vi "HFRR ADV v10.vi"() -> ()   [LabVIEW 2025]
uses:
  <vilib>/picture/picture.llb/imagedata.ctl
  src/Support Vi/Auto Start enum.ctl
  src/CAMERA CODE/CAMERA LIVE FEED ENUM.ctl
  src/CAMERA CODE/POST ANALYSIS ENUM.ctl
  <vilib>/Utility/NIReport.llb/HTML Report Image Alignment.ctl
  9464fbe3-7a28-44f6-aba5-8c8738b059c4.vi
  65798b11-504e-4bc8-a248-6a605d2bfeff.vi
  e8a7d01f-49de-42c3-94d4-2c8624f58f4e.vi
  5efb8110-29bd-47d9-92d0-c4703c9d257e.vi
  <vilib>/Analysis/baseanly.llb/Mean (DBL).vi
  <vilib>/Analysis/5stat.llb/RMS (DBL).vi
  c311699a-12ba-46ef-ac8f-427021fdbf06.vi
  b1c79803-6f73-4462-b675-f7b5eb88be7c.vi
  62610586-f3e3-47d7-ba3d-7d74a0c80884.vi
  25e8caaf-84ea-468e-9ff7-adb0e8b96af1.vi
  63a25930-3a94-42f5-b8a7-a5485c4ba60b.vi
  865355ac-209e-4fc1-945d-f9c41f79343a.vi
  8bf3357a-fd86-4b15-a53b-ddd460c8ef7b.vi
  8955922f-f541-41b3-8336-ee15e0ce1609.vi
  <vilib>/Analysis/4window.llb/Hanning Window (DBL).vi
  <vilib>/Utility/error.llb/Trim Whitespace One-Sided.vi
  <vilib>/Analysis/4window.llb/AllCosWindow (DBL).vi
  Instance          27 41Saved   WinDucom--std ed hfrr-WO 2464 v02 .vi
  <vilib>/Instr/_visa.llb/VISA Configure Serial Port (Instr).vi
  Instance          17 41Saved   WinDucom--std ed hfrr-WO 2464 v02 .vi
  Instance          37 41Saved   WinDucom--std ed hfrr-WO 2464 v02 .vi
  Instance          15 41Saved   WinDucom--std ed hfrr-WO 2464 v02 .vi
  <vilib>/addons/control/pid/pid.llb/PID (DBL).vi
  Instance          20 41Saved   WinDucom--std ed hfrr-WO 2464 v02 .vi
  <vilib>/measure/matone.llb/Extract Single Tone Information 1 Chan.vi
  Instance          10 41Saved   WinDucom--std ed hfrr-WO 2464 v02 .vi
  Instance          23 41Saved   WinDucom--std ed hfrr-WO 2464 v02 .vi
  <vilib>/Utility/NIReport.llb/Append Image to Report (path wrap).vi
  <vilib>/printing/OpenHTMLReport.llb/Open HTML Report in Browser (Refnum).vi
  <vilib>/Utility/NIReport.llb/Append Report Text (str wrap).vi
  Instance          11 41Saved   WinDucom--std ed hfrr-WO 2464 v02 .vi
  Instance           6 41Saved   WinDucom--std ed hfrr-WO 2464 v02 .vi
  Instance          28 41Saved   WinDucom--std ed hfrr-WO 2464 v02 .vi
  <vilib>/Utility/NIReport.llb/NI_report.lvclass
  <vilib>/addons/control/pid/NI_PID_pid.lvlib
  <vilib>/measure/NI_MAPro.lvlib
  <vilib>/ptbypt/NI_PtbyPt.lvlib
  Instance          22 41Saved   WinDucom--std ed hfrr-WO 2464 v02 .vi
  Instance          25 41Saved   WinDucom--std ed hfrr-WO 2464 v02 .vi
  <vilib>/NI Modbus.llb/MB Serial Master Query Read Input Registers (poly).vi
  Instance          35 41Saved   WinDucom--std ed hfrr-WO 2464 v02 .vi
  Instance          38 41Saved   WinDucom--std ed hfrr-WO 2464 v02 .vi
  <vilib>/measure/NI_MABase.lvlib
  <vilib>/Utility/NIReport.llb/NI_ReportGenerationCore.lvlib
  <vilib>/Analysis/NI_AALPro.lvlib
  <vilib>/Analysis/NI_AALBase.lvlib
  kernel32.dll
  <vilib>/NI Modbus.llb/MB Serial Master Query Write Single Register (poly).vi
panel:
  out "ELAPSED INDICATION":bool
  in  "main tab sub":enum32{"Page 1", "Page 2"}(tab)
  out "About":cluster{"About Display":string}={"About Display"="Software Version : Lab IQ\\WO 2465\\ v10\n\nRelease Period    : April 2026  "}
  in  "Info":bool
  in  "Quit":bool
  out "Humidity Port":bool=TRUE caption="Port 2"
  out "Standard 2":string="ASTM D6079 TEST CONDITIONS"
  out "powstat":bool caption="Power Status"
  out "Test \nStatus":bool caption="Test Status"
  out "Port 3":bool=TRUE caption="Port 1"
  out "Port 1a":bool caption="Port 1 a"
  out "Port 4":bool=TRUE caption="Port 2"
  out "Port 2a":bool caption="Port 2 a"
  in  "Main Dashboard Buttons":T1(radio) caption="Radio Buttons - Customizable"
  out "Time Stamp":string
  in  "Main Tab":T2(tab)
  out "Service Password Log":string="Incorrect Password"
  in  "Password 3":cluster{"Service Password":string}
  in  "Headen Service Button":bool
  in  "Sign In":bool
  in  "USER ID":string
  in  "USERNAME":string
  out "Auto Scar Check":cluster{"String 2":string}
  in  "Calibration":bool
  in  "Auto":bool
  in  "test time":dbl=75.0 caption="TEST DURATION" min=1.0 max=75.0 step=1.0
  in  "Set Rh":dbl=53.0 caption="HUMIDITY" min=53.0 max=53.0 step=1.0
  in  "Set Temp":dbl=60.0 caption="TEMPERATURE" min=40.0 max=150.0 step=1.0
  in  "Set Strk":dbl=1.0 caption="STROKE LENGTH" min=1.0 max=1.0 step=1.0 format="%.3f"
  in  "NORMAL LOAD":dbl=2.0 caption="APPLIED LOAD" min=1.0 max=10.0 step=1.0
  in  "Set Hz":dbl=50.0 caption="FREQUENCY" min=50.0 max=50.0 step=50.0 format="%.1f"
  out "Standard":string="ASTM D6079 TEST CONDITIONS"
  in  "FILE":string caption="FILE NAME"
  in  "Fuel Discription :":string caption="FLUID DESCRIPTION"
  in  "Batch Ref Num :":string caption="BATCH REF NO"
  in  "Remarks :":string caption="REMARKS"
  in  "tested by":string caption="TESTED BY"
  in  "Operator ID":string caption="OPERATOR ID"
  in  "TEST STANDARD":T3(ring)
  in  "Save & Continue":bool
  in  "Calibration 2":enum32{"Main", "Page 2"}(tab)
  in  "Cal Password":string
  out "Wrong Password":string="Wrong Password Entered"
  out "Time Remaining":dbl min=0.0 max=6000.0 step=0.01 format="%<%M:%S>t"
  in  "EVENT LOG":string="4:36:36 PM       Temperature trip enabled\n4:59:03 PM       Test started  — ASTM D6079-25"
  in  "Single/Multiple":enum32{"Single ", "Multiple"}(radio)=enum."Multiple" caption="Radio Buttons - Customizable"
  in  "Single - Graph":u16(ring) items=["Co-efficient of Friction", "Frictional Force ( N )", "ECR ( % )", "Temperature ( Deg C )", "Humidity ( %RH )", "Stroke ( mm )"]
  in  "Num/Graph":enum32{"Numeric Display", "Graph Display"}(radio) caption="Radio Buttons - Customizable"
  in  "Reset Graph":bool
  in  "Main Tab Display":T4(tab)
  in  "FRICVALZ 4":bool
  out "Set Stroke:":dbl
  out "Set Frequency:":dbl
  out "Set Humidity:":dbl
  out "Set Temperature:":dbl
  in  "Humidity":bool
  out "Horizontal Slider Control":dbl(slide) min=0.0 max=100.0 scale=0.0..75.0
  in  "Heater Button":bool
  out "HEATER":bool
  out "Humidity ( %RH )":dbl caption="Humidity 3" format="%.1f"
  out "AIR TEMP":dbl caption="Air Temperature  ( °C )" min=0.0 max=150.0 step=1.0 format="%.1f"
  out "Frequency ( Hz )":dbl=50.0 caption="Frequency" min=10.0 max=250.0 step=0.1 format="%.1f"
  out "Stroke 2":dbl=1.0 caption="Stroke" format="%.3f"
  out "Stroke":dbl=-1.7485910993892546e-16 format="%.3f"
  out "TEMP":dbl min=0.0 max=150.0 step=1.0 format="%.1f"
  out "ecr 3":dbl min=0.0 max=100.0 step=1.0
  out "FF 3":dbl min=0.0 max=12.0 step=0.01 format="%.3f"
  out "COF 3":dbl min=0.0 max=1.0 step=0.001 format="%.3f"
  in  "Ambient Humidity :":dbl format="%.1f"
  out "Hum":dbl=34.66389660208565 min=0.0 max=150.0 step=1.0
  out "Stroke 4":dbl=1.0 caption="Stroke" format="%.3f"
  out "Stroke ( mm )":cluster{"y":dbl, dbl, "y":dbl}(graph) caption="Waveform Chart - Light"
  out "Humidity ( %RH )":dbl(graph) caption="Waveform Chart - Light"
  out "Status 13":bool
  in  "Set Temp 2":dbl=65.0 caption="TRIP" min=20.0 max=150.0 step=1.0
  in  "trip1 8":bool
  in  "FRICVALZ 2":bool
  out "COF 2":dbl min=0.0 max=1.0 step=0.001 format="%.3f"
  out "Coefficient of Friction":dbl(graph) caption="Waveform Chart - Light"
  out "ecr":dbl min=0.0 max=100.0 step=1.0
  out "Electrical Contact Resistance ( % )":dbl(graph) caption="Waveform Chart - Light"
  out "FF 2":dbl min=0.0 max=12.0 step=0.01 format="%.3f"
  out "Frictional Force ( N )":dbl(graph) caption="Waveform Chart - Light"
  out "TEMP 2":dbl=34.66389660208565 min=0.0 max=150.0 step=1.0
  out "Temperature ( Deg C )":dbl(graph) caption="Waveform Chart - Light"
  out "Single":T5(tab)
  out "COF 4":dbl min=0.0 max=1.0 step=0.001 format="%.3f"
  out "Coefficient of Friction":dbl(graph) caption="Waveform Chart - Light"
  out "FF 4":dbl min=0.0 max=12.0 step=0.01 format="%.3f"
  in  "FRICVALZ 3":bool
  out "Frictional Force ( N )":dbl(graph) caption="Waveform Chart - Light"
  out "ecr 4":dbl min=0.0 max=100.0 step=1.0
  out "Electrical Contact Resistance ( % )":dbl(graph) caption="Waveform Chart - Light"
  out "TEMP 3":dbl=34.66389660208565 min=0.0 max=150.0 step=1.0
  out "Temperature ( Deg C )":dbl(graph) caption="Waveform Chart - Light"
  out "Hum 2":dbl=34.66389660208565 min=0.0 max=150.0 step=1.0
  out "Humidity ( %RH )":dbl(graph) caption="Waveform Chart - Light"
  out "Stroke 3":dbl=1.0 caption="Stroke" format="%.3f"
  out "Stroke ( mm )":cluster{"y":dbl, dbl, "y":dbl}(graph) caption="Waveform Chart - Light"
  out "Test Duration Display":string
  in  "Test Duration Status":dbl(slide) scale=0.0..100.0
  in  "RUN":bool
  in  "Auto Start Test":bool caption="RUN"
  out "Auto Scar Check  2":cluster{"String 2":string}
  in  "Magnification len live scar":string(combo)="5x" caption="MAGNIFICATION LEVEL"
  in  "FILE 3":string(combo) caption="FILE NAME"
  in  "SCAR MEASURMENT":enum32{"Auto Scar", "Manual Scar"}(radio)=enum."Manual Scar" caption="Radio Buttons - Customizable"
  in  "Cap Live Image":bool caption="Save Image"
  out "Zoom Factore":dbl format="%#.0f"
  in  "OUT":bool
  in  "In":bool
  in  "Confirm Measrurement":bool
  in  "Magnification :":string(combo)="5x"
  in  "Open Image":bool
  in  "Test File List :":string(combo)
  in  "Calibration Tab":enum32{"Measrument", "Calibrate"}(tab)
  out "Major Axis":dbl
  out "Minor Axis":dbl
  out "Average":dbl
  in  "Back Square":bool
  out "10x Gain":dbl
  out "5x Gain":dbl
  in  "Actual (µm)":dbl=1.0 caption="Actual (mm)" format="%.6f"
  out "Measurment (mm)":dbl caption="mm" format="%.3f"
  in  "Save Change":bool caption="Save Cal"
  in  "change Gain":bool
  in  "Calibrate":bool
  in  "Resize Tool":bool
  in  "Fit to Screen Tool":bool
  in  "ROI Color Tool":bool
  in  "Clear ROI Tool":bool
  in  "Rectangle Tool":bool
  in  "Pan Tool":bool
  in  "line tool":bool
  in  "Frequency":bool
  in  "Sample Temperature":bool
  in  "Stroke":bool
  in  "Humidity":bool
  in  "Air Temperature":bool
  in  "Tab Control 2":T6(tab)=enum."Humidity"
  in  "rstv2":bool
  out "Coefficient Of Friction":cluster{dbl[], dbl[]}[](graph)
  out "КОФ1":dbl caption="COF1 :" min=0.0 max=200.0 step=0.1 format="%.3f"
  out "КОФ2":dbl caption="COF2 :" min=0.0 max=200.0 step=0.1 format="%.3f"
  out "КОФ3":dbl caption="COF3 :" min=0.0 max=200.0 step=0.1 format="%.3f"
  out "КОФ4":dbl caption="COF4 :" min=0.0 max=200.0 step=0.1 format="%.3f"
  in  "RSTV1 3":bool
  out "Air Temperature  ( °C )":cluster{dbl[], dbl[]}[](graph)
  in  "RSTV1 2":bool
  out "Humidity ( %RH )":cluster{dbl[], dbl[]}[](graph)
  in  "RSTV1 4":bool
  out "Stroke ( mm )":cluster{dbl[], dbl[]}[](graph)
  out "КОФ2 5":dbl caption="Stroke 4 :" min=0.0 max=200.0 step=0.1 format="%.3f"
  out "КОФ2 4":dbl caption="Stroke 3 :" min=0.0 max=200.0 step=0.1 format="%.3f"
  out "КОФ2 3":dbl caption="Stroke 2 :" min=0.0 max=200.0 step=0.1 format="%.3f"
  out "КОФ2 2":dbl caption="Stroke 1:" min=0.0 max=200.0 step=0.1 format="%.3f"
  out "CP2":dbl=nan min=0.0 max=200.0 step=0.1 format="%.3f"
  out "CP1":dbl=nan min=0.0 max=200.0 step=0.1 format="%.3f"
  in  "RST CP":bool
  out "Sample Temperature ( °C )":cluster{dbl[], dbl[]}[](graph)
  in  "RST CP 2":bool
  out "XY Graph 13":cluster{dbl[], dbl[]}[](graph)
  out "Frequency ( Hz )":cluster{dbl[], dbl[]}[](graph)
  in  "RST CP 3":bool
  out "Air Temp ( °C ) vs Humidity ( % RH )":cluster{dbl[], dbl[]}[](graph)
  in  "OPEN 1":bool
  out "String Control 2":string="  "
  out "String Control":string
  out "String Control 7":string
  in  "OPEN 4":bool
  out "String Control 8":string=" "
  in  "OPEN 2":bool
  out "String Control 3":string
  out "String Control 4":string=" "
  in  "OPEN 3":bool
  out "String Control 6":string=" "
  out "String Control 5":string
  in  "Coefficient Of Friction":bool
  in  "OPEN":bool
  in  "Tab Control 5":T7(tab)
  in  "message":string="*Entered password is wrong"
  in  "Password 2":string caption="Password (Advance Setting)"
  in  "EDIT 2":bool
  in  "Language Selection":enum16{"English", "Russian"}(ring)
  in  "SrvM CP 2":bool caption="Reset calibrate\n password"
  in  "SrvM CP":bool caption="Reset calibrate\n password"
  in  "Password":string
  in  "SAVE":bool
  in  "File Path":path=path "C:/LAB-IQ-NXT 2010/1582/1582" caption="File path"
  in  "EDIT":bool
  out "AIR TEMPERATURE  Calibration Error":dbl=1.0 caption="Air Temperature :" min=0.0001 max=100.0 step=0.0001
  out "TEMPERATURE  Calibration Error":dbl=1.0 caption="Temperature :" min=0.0001 max=100.0 step=0.0001
  out "HUMIDITY  Calibration Error":dbl=1.0 caption="Humidity :"
  out "DISPLACEMENT  Calibration Error":dbl=1.0255 caption="Displacement :"
  out "STROKE Calibration Error":dbl=700.0 caption="Stroke Gain :"
  out "FRIC. FORCE Calibration Error":dbl=3.7633 caption="Frictional Force :" min=0.0001 max=100.0 step=0.0001
  in  "AIR TEMP INTERCEPT: 2":dbl=-2.9906 caption="Air Temperature Intercept:" format="%.4f"
  in  "AIR TEMP INTERCEPT:":dbl caption="Air Temperature Intercept :" format="%.4f"
  in  "TEMP INTERCEPT: 2":dbl=-2.9906 caption="Temperature Intercept :" format="%.4f"
  in  "TEMP INTERCEPT:":dbl caption="Temperature Intercept :" format="%.4f"
  in  "AIR TEMPERATURE : 2":dbl=57.9984 caption="Air Temperature :" min=0.0001 max=100.0 step=0.0001 format="%.4f"
  in  "AIR TEMPERATURE :":dbl=1.0 caption="Air Temperature :" min=0.0001 max=100.0 step=0.0001 format="%.4f"
  in  "TEMPERATURE : 2":dbl=57.9984 caption="Temperature :" min=0.0001 max=100.0 step=0.0001 format="%.4f"
  in  "TEMPERATURE :":dbl=1.0 caption="Temperature :" min=0.0001 max=100.0 step=0.0001 format="%.4f"
  in  "HUMIDITY: 2":dbl=1.0 caption="Humidity :" min=0.95 max=1.05 step=0.001 format="%.2f"
  in  "HUMIDITY:":dbl=1.0 caption="Humidity :" min=0.95 max=1.05 step=0.01 format="%.2f"
  in  "DISPLACEMENT : 4":dbl=0.88 caption="Displacement :" min=0.5 max=1.8 step=0.01 format="%#.2f"
  in  "DISPLACEMENT :":dbl=1.0255 caption="Displacement :"
  in  "STROKE GAIN : 2":dbl=900.0 caption="Stroke Gain :" min=500.0 max=1500.0 format="%#.1f"
  in  "STROKE GAIN :":dbl=700.0 caption="Stroke Gain :"
  in  "FRIC. FORCE : 2":dbl=1.0 caption="Frictional Force :" min=0.95 max=1.05 step=0.0001 format="%.2f"
  in  "FRIC. FORCE :":dbl=3.7633 caption="Frictional Force :" min=0.0001 max=100.0 step=0.0001 format="%.4f"
  in  "Tab Control 7":T8(tab)
  out "software msrnt 2":dbl=50.0 caption="Sensor measurment" min=0.0 max=250.0 step=0.001 format="%.4f"
  in  "S.NO":string="1333"
  out "DISPLACEMENT : 3":dbl=1.0255 caption="Corrected  gain:" format="%_2g"
  in  "DISPLACEMENT : 2":dbl=1.0 caption="Displacement  gain:" format="%_3g"
  in  "Standard Slip Gauge (mm)":dbl
  out "String 26":string="Rh"
  out "String 13":string="Rh"
  out "String 5":string="N"
  out "String 3":string="Hz"
  out "Time slide":dbl(slide)=70.0 scale=0.0..2500.0
  in  "Threshold":dbl=0.2 min=0.0 max=5.0 step=0.001 format="%.3f"
  out "Lift":bool
  out "FF Calibration g":dbl[](graph)=[-0.1159806317003227, -0.11422308310659272, -0.10192024295047254, -0.10719288873166506, -0.09840514576301, -0.1036777915442051, -0.09489004857554746, -0.08961740279435236, -0.10192024295047254, -0.09664759716928002, -0.08785985420062238, -0.08785985420062238, -0.08434475701316244, -0.0755570140445048, -0.07204191685704484, -0.07204191685704484, -0.0808296598256999, -0.07379946545077481, -0.07379946545077481, -0.0755570140445048, -0.07379946545077481, -0.07204191685704484, -0.0755570140445048, -0.07028436826331227, -0.07379946545077481, -0.07379946545077481, -0.0685268196695823, 0.014077964235786087, -0.02458810482629926, -0.05270888232599699, -0.0632541738883872, -0.059739076700924654, -0.07379946545077481, -0.0755570140445048, -0.06501172248211717, -0.0685268196695823, -0.06501172248211717, -0.0632541738883872, -0.07028436826331227, -0.06501172248211717, -0.06149662529465463, -0.05622397951346211, -0.05622397951346211, -0.05622397951346211, -0.054466430919732134, -0.054466430919732134, -0.04919378513853445, -0.04392113935734194, -0.04743623654480447, -0.04392113935734194, -0.04392113935734194, -0.03689094498241944, -0.028103202013764383, -0.02107300763883672, -0.02107300763883672, -0.017557910451374184, -0.017557910451374184, -0.010527716076451686, -0.008770167482716543, -0.008770167482716543, -0.008770167482716543, -0.007012618888986565, -0.0017399731077940475, 0.001775124079668492, 0.007047769860861009, 0.012320415642053526, 0.019350610016981188, 0.029895901579366224, 0.036926095954293886, 0.033410998766831346, 0.033410998766831346, 0.036926095954293886, 0.04395629032921638, 0.05098648470414146, 0.05625913048533398, 0.06504687345399161, 0.06856197064145415, 0.0773497136101118, 0.09316765095369194, 0.08789500517249683, 0.09844029673488704, 0.10195539392234698, 0.10722803970354466, 0.11074313689100462, 0.11425823407846716, 0.11425823407846716, 0.12656107423458476, 0.1353488172032424, 0.14413656017189747, 0.1546818517342851, 0.16171204610921017, 0.16874224048413264, 0.1652271432966701, 0.1757724348590603, 0.17752998345279028, 0.18983282360890788, 0.18983282360890788, 0.19862056657756552, 0.20389321235875804, 0.21092340673368312, 0.22146869829607074, 0.22674134407726326, 0.22146869829607074, 0.22498379548353328, 0.2302564412647258, 0.2355290870459209, 0.24080173282711342, 0.24783192720204109, 0.24783192720204109, 0.254862121576961, 0.26189231595188867, 0.26892251032681375, 0.26892251032681375, 0.27419515610800627, 0.2777102532954714, 0.28474044767039386, 0.2900130934515864, 0.29177064204532155, 0.30758857938889905, 0.3058310307951691, 0.3128612251700916, 0.3251640653262118, 0.3234065167324818, 0.33746690548233194, 0.3304367111074043, 0.335709356888602, 0.41304149501277265, 0.3603150372008346, 0.35679994001337206, 0.35504239141964206, 0.3638301343882997, 0.36734523157576227, 0.4165565922002352, 0.45698020985605314, 0.4710405986059007, 0.47279814719963065, 0.4815858901682883, 0.4833434387620183, 0.5114642162617212, 0.4938887303244085, 0.4235867865751603, 0.39546600907546, 0.3884358147005323, 0.3884358147005323, 0.38667826610680234, 0.3919509118879974, 0.39546600907546, 0.4007386548566525, 0.3989811062629225, 0.4007386548566525, 0.40601130063784757, 0.40776884923158013, 0.4112839464190401, 0.4183141407939652, 0.42007168938769773, 0.42534433516889286, 0.4306169809500828, 0.43764717532500785, 0.44467736969993293, 0.4552226612623206, 0.4552226612623206, 0.4552226612623206, 0.4552226612623206, 0.45698020985605314, 0.4657679528247108, 0.4587377584497831, 0.45698020985605314, 0.4622528556372482, 0.4604953070435131, 0.4587377584497831, 0.47279814719963065, 0.4640104042309782, 0.4657679528247108, 0.46928305001217074, 0.4780707929808258, 0.4780707929808258, 0.47631324438709577, 0.4780707929808258, 0.47982834157455834, 0.48510098735575086, 0.49037363313694593, 0.49213118173067594, 0.49564627891813845, 0.5061915704805287, 0.5079491190742587, 0.5184944106366437, 0.5167368620429111, 0.5114642162617212, 0.5097066676679887, 0.5149793134491786, 0.5079491190742587, 0.5114642162617212, 0.5132217648554511, 0.5149793134491786, 0.5202519592303763, 0.5202519592303763, 0.5255246050115687, 0.5272821536053013, 0.5272821536053013, 0.5395849937614215, 0.536069896573959, 0.536069896573959, 0.5395849937614215, 0.5395849937614215, 0.5431000909488815, 0.5431000909488815, 0.5483727367300766, 0.553645382511269, 0.5501302853238066, 0.5483727367300766, 0.5483727367300766, 0.5518878339175392, 0.5501302853238066, 0.5501302853238066, 0.5606755768861942, 0.5571604796987316, 0.5641906740736593, 0.5589180282924616, 0.5571604796987316, 0.553645382511269, 0.5554029311050016, 0.5571604796987316, 0.5641906740736593, 0.5659482226673893, 0.5659482226673893, 0.5659482226673893, 0.5659482226673893, 0.5729784170423143, 0.5764935142297769, 0.5782510628235095, 0.5747359656360443, 0.5800086114172394, 0.5782510628235095, 0.5782510628235095, 0.5764935142297769, 0.5817661600109719, 0.5852812571984319, 0.592311451573357, 0.5993416459482795, 0.6098869375106697, 0.696006818603498, 0.7223700475094658, 0.6397652636040975, 0.6327350692291749, 0.6221897776667898, 0.6221897776667898, 0.6274624234479824, 0.6221897776667898, 0.6327350692291749, 0.6380077150103675, 0.6432803607915599, 0.64152281219783, 0.64152281219783, 0.6520681037602176, 0.6590982981351426, 0.6590982981351426, 0.6573407495414101, 0.6573407495414101, 0.6590982981351426, 0.6608558467288727, 0.6696435896975302, 0.6573407495414101, 0.6608558467288727, 0.6696435896975302, 0.6714011382912628, 0.6731586868849928, 0.6766737840724554, 0.6801888812599153, 0.6784313326661854, 0.6766737840724554, 0.6819464298536478, 0.6784313326661854, 0.6784313326661854, 0.6749162354787203, 0.6749162354787203, 0.6749162354787203, 0.6749162354787203, 0.6784313326661854, 0.6837039784473778, 0.6819464298536478, 0.6819464298536478, 0.6854615270411104, 0.6837039784473778, 0.6784313326661854, 0.6784313326661854, 0.6749162354787203, 0.6784313326661854, 0.6784313326661854, 0.6714011382912628, 0.6696435896975302, 0.6696435896975302, 0.6626133953226078, 0.6714011382912628, 0.6608558467288727, 0.6538256523539502, 0.6520681037602176, 0.6538256523539502, 0.6503105551664876, 0.6555832009476801, 0.6590982981351426, 0.6626133953226078, 0.6643709439163378, 0.6608558467288727, 0.6590982981351426, 0.6520681037602176, 0.6432803607915599, 0.6432803607915599, 0.6538256523539502, 0.6467954579790225, 0.6450379093852925, 0.6450379093852925, 0.6450379093852925, 0.64152281219783, 0.6432803607915599, 0.64152281219783, 0.6380077150103675, 0.6362501664166375, 0.6344926178229049, 0.6344926178229049, 0.6362501664166375, 0.6362501664166375, 0.64152281219783, 0.6432803607915599, 0.6450379093852925, 0.6520681037602176, 0.6520681037602176, 0.648553006572755, 0.6538256523539502, 0.6538256523539502, 0.6590982981351426, 0.6643709439163378, 0.6696435896975302, 0.6837039784473778, 0.6872190756348404, 0.6924917214160355, 0.697764367197228, 0.6924917214160355, 0.6942492700097681, 0.7100672073533482, 0.7698238595402062, 0.7311577904781209, 0.7223700475094658, 0.7223700475094658, 0.7241275961031958, 0.7294002418843883, 0.7733389567276687, 0.8330956089145345, 0.8278229631333368, 0.8418833518831895, 0.8506710948518446, 0.8664890321954247, 0.8717616779766173, 0.8893371639139299, 0.9016400040700475, 0.9121852956324352, 0.9280032329760178, 0.9139428442261678, 0.9139428442261678, 0.9157003928198977, 0.9227305871948254, 0.9543664618819856, 0.9561240104757156, 0.9420636217258654, 0.9789721421942235, 0.9543664618819856, 0.9666693020381032, 0.980729690787956, 0.9666693020381032, 0.892852261101395, 0.8787918723515449, 0.8840645181327375, 0.8823069695390074, 0.8858220667264675, 0.8875796153202, 0.8875796153202, 0.8840645181327375, 0.8893371639139299, 0.8893371639139299, 0.8981249068825851, 0.8981249068825851, 0.8981249068825851, 0.8981249068825851, 0.9051551012575126, 0.9051551012575126, 0.9192154900073628, 0.9104277470387052, 0.9139428442261678, 0.9192154900073628, 0.9244881357885554, 0.9227305871948254, 0.9209730386010928, 0.9280032329760178, 0.9297607815697478, 0.933275878757213, 0.9367909759446755, 0.9385485245384029, 0.9367909759446755, 0.9403060731321329, 0.9438211703195954, 0.9543664618819856, 0.9420636217258654, 0.9473362675070606, 0.9473362675070606, 0.9490938161007906, 0.9490938161007906, 0.9473362675070606, 0.9473362675070606, 0.9508513646945231, 0.9543664618819856, 0.9596391076631782, 0.9578815590694456, 0.9613966562569107, 0.9631542048506433, 0.9719419478192983, 0.9754570450067583, 0.980729690787956, 0.9877598851628785, 0.9877598851628785, 0.9877598851628785, 0.9947900795378062, 0.9965476281315361, 0.9912749823503436, 0.989517433756611, 0.9983051767252686, 1.0018202739127287, 1.0053353711001938, 1.0088504682876562, 1.0123655654751162, 1.0211533084437738, 1.0158806626625763, 1.0193957598500414, 1.0281835028186963, 1.0229108570375038, 1.0246684056312338, 1.0281835028186963, 1.0281835028186963, 1.0281835028186963, 1.035213697193624, 1.035213697193624, 1.0369712457873541, 1.0334561485998914, 1.0404863429748166, 1.045758988756009, 1.0369712457873541, 1.0334561485998914, 1.0404863429748166, 1.031698600006159, 1.0334561485998914, 1.0387287943810866, 1.0404863429748166, 1.0422438915685466, 1.044001440162279, 1.1195760296927224, 1.1371515156300351, 1.0580618289121266, 1.0510316345372042, 1.0387287943810866, 1.0387287943810866, 1.0369712457873541, 1.031698600006159, 1.0404863429748166, 1.0404863429748166, 1.044001440162279, 1.045758988756009, 1.045758988756009, 1.045758988756009, 1.0510316345372042, 1.045758988756009, 1.0422438915685466, 1.0422438915685466, 1.0387287943810866, 1.0334561485998914, 1.0369712457873541, 1.0387287943810866, 1.031698600006159, 1.0387287943810866, 1.029941051412429, 1.0404863429748166, 1.031698600006159, 1.0334561485998914, 1.035213697193624, 1.0369712457873541, 1.0334561485998914, 1.0334561485998914, 1.0527891831309368, 1.0422438915685466, 1.035213697193624, 1.0334561485998914, 1.029941051412429, 1.0264259542249663, 1.0281835028186963, 1.0211533084437738, 1.0264259542249663, 1.0158806626625763, 1.0158806626625763, 1.0176382112563087, 1.0106080168813836, 1.0088504682876562, 1.0088504682876562, 1.0070929196939262, 1.0070929196939262, 1.0123655654751162, 1.0123655654751162, 1.0158806626625763, 1.0158806626625763, 1.0176382112563087, 1.0229108570375038, 1.0141231140688463, 1.0158806626625763, 1.0193957598500414, 1.0176382112563087, 1.0176382112563087, 1.0193957598500414, 1.0229108570375038, 1.0264259542249663, 1.0229108570375038, 1.031698600006159, 1.0264259542249663, 1.0334561485998914, 1.0369712457873541, 1.0422438915685466, 1.0527891831309368, 1.0492740859434742, 1.0492740859434742, 1.0545467317246642, 1.0563042803183942, 1.0615769260995918, 1.0650920232870518, 1.070364669068247, 1.0756373148494394, 1.084425057818097, 1.091455252193022, 1.0949703493804845, 1.102000543755407, 1.1090307381303321, 1.1195760296927224, 1.117818481098987, 1.1230911268801824, 1.1301213212551073, 1.1266062240676449, 1.1248486754739149, 1.1318788698488373, 1.1371515156300351, 1.1512119043798827, 1.1512119043798827, 1.1547270015673425, 1.1599996473485377, 1.1705449389109253, 1.1740600360983877, 1.1723024875046555, 1.175817584692118, 1.179332681879583, 1.2320591396915157, 1.2144836537542059, 1.2426044312539035, 1.2900582432846492, 1.3006035348470342, 1.3076337292219617, 1.3287243123467318, 1.3656328328150897, 1.3691479300025498, 1.37969322156494, 1.3779356729712073, 1.388480964533595, 1.39375361031479, 1.402541353283445, 1.4095715476583677, 1.4130866448458301, 1.4183592906270253, 1.4078139990646377, 1.4166017420332928, 1.402541353283445, 1.4060564504709077, 1.420116839220758, 1.4183592906270253, 1.4113290962521003, 1.4218743878144877, 1.420116839220758, 1.3867234159398627, 1.36739038140882, 1.3621177356276275, 1.3586026384401648, 1.3709054785962824, 1.36739038140882, 1.36739038140882, 1.36739038140882, 1.36739038140882, 1.3656328328150897, 1.36739038140882, 1.3638752842213573, 1.3603601870338946, 1.3515724440652397, 1.3515724440652397, 1.3410271525028519, 1.3375120553153894, 1.332239409534197, 1.3269667637530018, 1.3216941179718094, 1.3234516665655394, 1.309391277815692, 1.2812705003159917, 1.2988459862533042, 1.3252092151592694, 1.3129063750031542, 1.3041186320344993, 1.3041186320344993, 1.3023610834407642, 1.293573340472109, 1.3041186320344993, 1.2953308890658417, 1.2847855975034512, 1.291815791878379, 1.291815791878379, 1.2900582432846492, 1.3006035348470342, 1.288300694690914, 1.2830280489097214, 1.2830280489097214, 1.2847855975034512, 1.2847855975034512, 1.288300694690914, 1.288300694690914, 1.2900582432846492, 1.2900582432846492, 1.291815791878379, 1.2988459862533042, 1.3006035348470342, 1.3006035348470342, 1.293573340472109, 1.288300694690914, 1.2988459862533042, 1.3006035348470342, 1.3023610834407642, 1.3023610834407642, 1.2970884376595715, 1.2953308890658417, 1.3006035348470342, 1.2988459862533042, 1.3006035348470342, 1.3076337292219617, 1.309391277815692, 1.309391277815692, 1.3164214721906167, 1.3287243123467318, 1.3287243123467318, 1.3269667637530018, 1.3287243123467318, 1.3410271525028519, 1.3445422496903146, 1.3515724440652397, 1.3533299926589721, 1.3621177356276275, 1.3621177356276275, 1.3656328328150897, 1.3744205757837422, 1.3744205757837422, 1.3709054785962824, 1.3744205757837422, 1.3761781243774776, 1.3779356729712073, 1.38145077015867, 1.3849658673461325, 1.3902385131273278, 1.3919960617210576, 1.3902385131273278, 1.4253894850019504, 1.420116839220758, 1.3304818609404645, 1.3146639235968844, 1.3146639235968844, 1.3129063750031542, 1.3146639235968844, 1.318179020784347, 1.318179020784347, 1.3216941179718094, 1.3252092151592694, 1.332239409534197, 1.3304818609404645, 1.3252092151592694, 1.3252092151592694, 1.319936569378077, 1.3216941179718094, 1.3216941179718094, 1.3216941179718094, 1.319936569378077, 1.319936569378077, 1.319936569378077, 1.318179020784347, 1.3146639235968844, 1.3234516665655394, 1.319936569378077, 1.3164214721906167, 1.3216941179718094, 1.319936569378077, 1.3146639235968844, 1.3164214721906167, 1.3164214721906167, 1.3164214721906167, 1.3357545067216594, 1.318179020784347, 1.3146639235968844, 1.3129063750031542, 1.3058761806282293, 1.3111488264094218, 1.3058761806282293, 1.3076337292219617, 1.3216941179718094, 1.3146639235968844, 1.3146639235968844, 1.3111488264094218, 1.3076337292219617, 1.3058761806282293, 1.3023610834407642, 1.3058761806282293, 1.3058761806282293, 1.3058761806282293, 1.3023610834407642, 1.2953308890658417, 1.3023610834407642, 1.3006035348470342, 1.2970884376595715, 1.2970884376595715, 1.2970884376595715, 1.2970884376595715, 1.2900582432846492, 1.2830280489097214, 1.2830280489097214, 1.2795129517222588, 1.275997854534799, 1.277755403128529, 1.275997854534799, 1.2707252087536038, 1.2689676601598738, 1.2689676601598738, 1.2707252087536038, 1.275997854534799, 1.2689676601598738, 1.2636950143786811, 1.2672101115661438, 1.2566648200037538, 1.2531497228162913, 1.249634625628831, 1.2478770770350986, 1.249634625628831, 1.2478770770350986, 1.246119528441366, 1.2408468826601735, 1.2408468826601735, 1.237331785472711, 1.2338166882852486, 1.2338166882852486, 1.2285440425040561, 1.219756299535401, 1.226786493910326, 1.2215138481291308, 1.219756299535401, 1.2215138481291308, 1.2179987509416683, 1.219756299535401, 1.2250289453165935, 1.226786493910326, 1.2303015910977835, 1.2320591396915157, 1.226786493910326, 1.226786493910326, 1.2303015910977835, 1.2636950143786811, 1.261937465784949, 1.2443619798476335, 1.2426044312539035, 1.239089334066441, 1.2408468826601735, 1.249634625628831, 1.3357545067216594, 1.332239409534197, 1.3445422496903146, 1.3586026384401648, 1.3709054785962824, 1.3761781243774776, 1.3972687075022525, 1.38145077015867, 1.3058761806282293, 1.293573340472109, 1.277755403128529, 1.2672101115661438, 1.2672101115661438, 1.2707252087536038, 1.275997854534799, 1.277755403128529, 1.2812705003159917, 1.2812705003159917, 1.288300694690914, 1.2900582432846492, 1.2900582432846492, 1.288300694690914, 1.2900582432846492, 1.2900582432846492, 1.2953308890658417, 1.293573340472109, 1.3058761806282293, 1.2988459862533042, 1.2988459862533042, 1.2988459862533042, 1.3006035348470342, 1.3041186320344993, 1.3146639235968844, 1.3076337292219617, 1.3076337292219617, 1.3076337292219617, 1.3058761806282293, 1.3058761806282293, 1.3129063750031542, 1.3146639235968844, 1.3164214721906167, 1.3287243123467318, 1.332239409534197, 1.332239409534197, 1.332239409534197, 1.332239409534197, 1.3269667637530018, 1.3304818609404645, 1.3269667637530018, 1.3252092151592694, 1.3304818609404645, 1.3287243123467318, 1.3287243123467318, 1.3357545067216594, 1.3357545067216594, 1.3410271525028519, 1.342784701096582, 1.3445422496903146, 1.3462997982840443, 1.3498148954715095, 1.3515724440652397, 1.3515724440652397, 1.3586026384401648, 1.3656328328150897, 1.3656328328150897, 1.3656328328150897, 1.3744205757837422, 1.3779356729712073, 1.3867234159398627, 1.388480964533595, 1.39375361031479, 1.3919960617210576, 1.3990262560959827, 1.3955111589085203, 1.3955111589085203, 1.3990262560959827, 1.3955111589085203, 1.3972687075022525, 1.3990262560959827, 1.4007838046897128, 1.4060564504709077, 1.4113290962521003, 1.4183592906270253, 1.4253894850019504, 1.4306621307831453, 1.4394498737518007, 1.4394498737518007, 1.4447225195329931, 1.4464800681267256, 1.449995165314188, 1.4552678110953834, 1.4552678110953834, 1.4570253596891134, 1.4570253596891134, 1.4587829082828432, 1.4587829082828432, 1.465813102657771, 1.4622980054703083, 1.4605404568765759, 1.4622980054703083, 1.4587829082828432, 1.4605404568765759, 1.4675706512515008, 1.4587829082828432, 1.4622980054703083, 1.464055554064041, 1.5343574978132866, 1.576538664062837, 1.4921763315637386, 1.4763583942201561, 1.4781159428138884, 1.4763583942201561, 1.472843297032696, 1.4693281998452334, 1.4693281998452334, 1.4675706512515008, 1.4710857484389634, 1.465813102657771, 1.4605404568765759, 1.4622980054703083, 1.4570253596891134, 1.4605404568765759, 1.464055554064041, 1.4675706512515008, 1.472843297032696, 1.4798734914076184, 1.4798734914076184, 1.4816310400013486, 1.485146137188811, 1.4833885885950808, 1.485146137188811, 1.4904187829700062, 1.4921763315637386, 1.4939338801574686, 1.499206525938661, 1.497448977344931, 1.499206525938661, 1.5027216231261236, 1.5079942689073187, 1.5027216231261236, 1.5027216231261236, 1.497448977344931, 1.495691428751201, 1.5009640745323938, 1.497448977344931, 1.5009640745323938, 1.5079942689073187, 1.5062367203135887, 1.523812206250899, 1.5202971090634363, 1.5220546576571663, 1.525569754844629, 1.525569754844629, 1.525569754844629, 1.5290848520320917, 1.5325999492195568, 1.5378725950007492, 1.539630143594479, 1.5431452407819417, 1.5484178865631366, 1.5519329837505993, 1.5589631781255242, 1.557205629531792, 1.565993372500447, 1.5624782753129893, 1.5607207267192542, 1.5624782753129893, 1.5589631781255242, 1.5624782753129893, 1.5624782753129893, 1.565993372500447, 1.5677509210941794, 1.5695084696879091, 1.5712660182816394, 1.5747811154691018, 1.5818113098440296, 1.585326407031492, 1.5888415042189519, 1.5958716985938797, 1.5976292471876095, 1.5993867957813424, 1.6029018929688048, 1.6029018929688048, 1.6011443443750721, 1.6046594415625373, 1.6064169901562673, 1.6064169901562673, 1.6081745387499973, 1.6064169901562673, 1.61520473312492, 1.61520473312492, 1.618719830312385, 1.62750757328104, 1.618719830312385, 1.618719830312385, 1.62926512187477, 1.6257500246873098, 1.6257500246873098, 1.6327802190622351, 1.63981041343716, 1.64156796203089, 1.6468406078120825, 1.6538708021870077, 1.6573858993744703, 1.6556283507807377, 1.6872642254679004, 1.6960519684365558, 1.6802340310929782, 1.6767189339055155, 1.6837491282804407, 1.6802340310929782, 1.6837491282804407, 1.782171849529389, 1.7804143009356566, 1.7892020439043117, 1.7997473354666966, 1.8102926270290869, 1.8155652728102794, 1.8208379185914743, 1.8173228214040091, 1.7259302945299884, 1.7048397114052134, 1.6960519684365558, 1.7101123571864059, 1.7048397114052134, 1.7013246142177483, 1.7065972599989456, 1.7083548085926759, 1.7101123571864059, 1.7136274543738683, 1.7171425515613308, 1.722415197342526, 1.7153850029676008, 1.7101123571864059, 1.7101123571864059, 1.7276878431237184, 1.7171425515613308, 1.7171425515613308, 1.7259302945299884, 1.7259302945299884, 1.741748231873566, 1.7364755860923762, 1.7364755860923762, 1.739990683279836, 1.739990683279836, 1.7382331346861086, 1.7435057804672986, 1.7329604889049162, 1.7329604889049162, 1.7259302945299884, 1.7136274543738683, 1.7101123571864059, 1.7083548085926759, 1.7083548085926759, 1.7083548085926759, 1.7171425515613308, 1.7065972599989456, 1.6960519684365558, 1.6960519684365558, 1.6942944198428282, 1.697809517030288, 1.6960519684365558, 1.6960519684365558, 1.6942944198428282, 1.697809517030288, 1.6925368712490982, 1.6942944198428282, 1.6960519684365558, 1.6890217740616331, 1.6872642254679004, 1.6942944198428282, 1.6837491282804407, 1.6872642254679004, 1.6837491282804407, 1.6802340310929782, 1.6784764824992453, 1.6907793226553656, 1.6855066768741707, 1.6802340310929782, 1.6767189339055155, 1.6749613853117828, 1.6767189339055155, 1.681991579686708, 1.681991579686708, 1.6942944198428282, 1.6890217740616331, 1.6855066768741707, 1.6960519684365558, 1.6925368712490982, 1.6925368712490982, 1.697809517030288, 1.7101123571864059, 1.7083548085926759, 1.7083548085926759, 1.7136274543738683, 1.7189001001550634, 1.7259302945299884, 1.7276878431237184, 1.734718037498646, 1.7329604889049162, 1.7312029403111808, 1.7329604889049162, 1.7382331346861086, 1.734718037498646, 1.7329604889049162, 1.7312029403111808, 1.7329604889049162, 1.734718037498646, 1.739990683279836, 1.7435057804672986, 1.7435057804672986, 1.7470208776547638, 1.7487784262484938, 1.757566169217149, 1.7540510720296862, 1.7558086206234187, 1.771626557966999, 1.7645963635920765, 1.7645963635920765, 1.824353015778937, 1.884109667965795, 1.7997473354666966, 1.7839293981231163, 1.7856869467168466, 1.787444495310579, 1.792717141091774, 1.787444495310579, 1.7804143009356566, 1.782171849529389, 1.7804143009356566, 1.7786567523419266, 1.787444495310579, 1.776899203748194, 1.782171849529389, 1.776899203748194, 1.776899203748194, 1.7804143009356566, 1.787444495310579, 1.792717141091774, 1.7909595924980442, 1.7997473354666966, 1.8050199812478944, 1.8050199812478944, 1.8102926270290869, 1.8120501756228167, 1.8173228214040091, 1.8208379185914743, 1.824353015778937, 1.831383210153857, 1.833140758747592, 1.833140758747592, 1.8366558559350545, 1.8401709531225146, 1.833140758747592, 1.834898307341322, 1.8436860503099772, 1.8366558559350545, 1.8384134045287848, 1.8366558559350545, 1.8384134045287848, 1.8472011474974424, 1.8436860503099772, 1.8507162446849048, 1.8595039876535597, 1.8542313418723673, 1.8612615362472924, 1.866534182028485, 1.8682917306222173, 1.866534182028485, 1.8682917306222173, 1.866534182028485, 1.8682917306222173, 1.8718068278096776, 1.8770794735908725, 1.8700492792159473, 1.8700492792159473, 1.87532192499714, 1.884109667965795, 1.884109667965795, 1.8876247651532576, 1.8893823137469927, 1.8911398623407227, 1.8893823137469927, 1.8946549595281854, 1.898170056715645, 1.898170056715645, 1.8964125081219152, 1.8999276053093779, 1.9016851539031077, 1.9052002510905728, 1.9052002510905728, 1.912230445465498, 1.9069577996843026, 1.9052002510905728, 1.9069577996843026, 1.912230445465498, 1.9052002510905728, 1.9034427024968403, 1.9034427024968403, 1.9016851539031077, 1.9016851539031077, 1.9069577996843026, 1.9104728968717652, 1.912230445465498, 1.9175030912466904, 1.9210181884341528, 1.9210181884341528, 1.913987994059228, 1.9175030912466904, 1.9333210285902707, 1.9227757370278828, 1.9280483828090755, 1.935078577184003, 1.9368361257777331, 1.935078577184003, 1.9473814173401207, 1.945623868746388, 1.9508965145275832, 1.9649569032774308, 1.991320132183401, 1.9596842574962356, 1.9544116117150456, 1.9491389659338532, 1.961441806089971, 1.9561691603087759, 2.049319235776529, 2.0458041385890664, 2.044046589995337, 2.0581069787451844, 2.0686522703075743, 2.0862277562448845, 2.079197561869962, 2.0528343329639918, 1.9825323892147435, 1.970229549058626, 1.9684720004648935, 1.973744646246086, 1.975502194839821, 1.9667144518711634, 1.9684720004648935, 1.975502194839821, 1.973744646246086, 1.973744646246086, 1.973744646246086, 1.973744646246086, 1.973744646246086, 1.971987097652356, 1.9790172920272835, 1.973744646246086, 1.975502194839821, 1.971987097652356, 1.9684720004648935, 1.971987097652356, 1.9667144518711634, 1.9667144518711634, 1.973744646246086, 1.9684720004648935, 1.971987097652356, 1.977259743433551, 1.971987097652356, 1.971987097652356, 1.9983503265583262, 1.977259743433551, 1.9790172920272835, 1.973744646246086, 1.9825323892147435, 1.9807748406210137, 1.9825323892147435, 1.9825323892147435, 1.9860474864022062, 1.977259743433551, 1.9807748406210137, 1.9842899378084762, 1.9842899378084762, 1.9825323892147435, 1.9842899378084762, 1.987805034995936, 1.9842899378084762, 1.9895625835896713, 1.9965927779645936, 1.9930776807771338, 1.9948352293708638, 1.9965927779645936, 2.0001078751520565, 2.0106531667144436, 2.0106531667144436, 2.0141682639019036, 2.017683361089369, 2.024713555464294, 2.026471104058024, 2.0335012984329515, 2.028228652651754, 2.028228652651754, 2.0335012984329515, 2.0352588470266815, 2.0370163956204115, 2.042289041401607, 2.042289041401607, 2.042289041401607, 2.0563494301514544, 2.0475616871827995, 2.0528343329639918, 2.0458041385890664, 2.044046589995337, 2.0458041385890664, 2.049319235776529, 2.0475616871827995, 2.0510767843702618, 2.0545918815577218, 2.0563494301514544, 2.0581069787451844, 2.066894721713842, 2.0616220759326493, 2.0563494301514544, 2.0563494301514544, 2.0510767843702618, 2.0563494301514544, 2.0475616871827995, 2.044046589995337, 2.0458041385890664, 2.044046589995337, 2.0370163956204115, 2.040531492807874, 2.0370163956204115, 2.0335012984329515, 2.0370163956204115, 2.0352588470266815, 2.0299862012454866, 2.0299862012454866, 2.028228652651754, 2.0352588470266815, 2.0352588470266815, 2.073924916088767, 2.135439116869365, 2.0686522703075743, 2.0510767843702618, 2.0475616871827995, 2.049319235776529, 2.0475616871827995, 2.044046589995337, 2.0475616871827995, 2.049319235776529, 2.0510767843702618, 2.0528343329639918, 2.0545918815577218, 2.0581069787451844, 2.049319235776529, 2.049319235776529, 2.0510767843702618, 2.0545918815577218, 2.0545918815577218, 2.0563494301514544, 2.0563494301514544, 2.0616220759326493, 2.066894721713842, 2.0633796245263794, 2.065137173120112, 2.0686522703075743, 2.079197561869962, 2.0827126590574245, 2.0827126590574245, 2.0862277562448845, 2.0932579506198095, 2.0879853048386168, 2.0915004020260795, 2.096773047807272, 2.096773047807272, 2.096773047807272, 2.1055607907759324, 2.103803242182197, 2.1055607907759324, 2.109075887963395, 2.119621179525782, 2.124893825306975, 2.1319240196819003, 2.135439116869365, 2.138954214056825, 2.1442268598380174, 2.14774195702548, 2.153014602806673, 2.153014602806673, 2.1600447971815977, 2.1670749915565253, 2.165317442962793, 2.165317442962793, 2.163559894369063, 2.1670749915565253, 2.1600447971815977, 2.1565296999941355, 2.1547721514004055, 2.153014602806673, 2.1547721514004055, 2.1618023457753304, 2.153014602806673, 2.1582872485878677, 2.1547721514004055, 2.1565296999941355, 2.1582872485878677, 2.1600447971815977, 2.1600447971815977, 2.165317442962793, 2.1705900887439857, 2.1705900887439857, 2.174105185931448, 2.1811353803063755, 2.1758627345251806, 2.1758627345251806, 2.1793778317126433, 2.1758627345251806, 2.1688325401502557, 2.163559894369063, 2.1618023457753304, 2.1565296999941355, 2.1547721514004055, 2.1459844084317505, 2.140711762650558, 2.137196665463095, 2.135439116869365, 2.142469311244288, 2.1336815682756325, 2.1319240196819003, 2.135439116869365, 2.1319240196819003, 2.142469311244288, 2.138954214056825, 2.135439116869365, 2.140711762650558, 2.1442268598380174, 2.1512570542129428, 2.153014602806673, 2.1547721514004055, 2.153014602806673, 2.1547721514004055, 2.195195769056223, 2.1547721514004055, 2.153014602806673, 2.1494995056192128, 2.1459844084317505, 2.1512570542129428, 2.233861838118314, 2.2215589979621937, 2.2268316437433864, 2.233861838118314, 2.2408920324932335, 2.2461646782744262, 2.2619826156180114, 2.2619826156180114, 2.2707703585866668, 2.2408920324932335, 2.2373769353057713, 2.242649581086964, 2.247922226868161, 2.2567099698368165, 2.228589192337116, 2.228589192337116, 2.2461646782744262, 2.1494995056192128, 2.1301664710881676, 2.119621179525782, 2.1161060823383173, 2.112590985150855, 2.1108334365571246, 2.1055607907759324, 2.100288144994735, 2.096773047807272, 2.100288144994735, 2.098530596401002, 2.103803242182197, 2.098530596401002, 2.0932579506198095, 2.1020456935884697, 2.0950154992135395, 2.0950154992135395, 2.0915004020260795, 2.0950154992135395, 2.0915004020260795, 2.103803242182197, 2.0879853048386168, 2.0879853048386168, 2.0844702076511545, 2.079197561869962, 2.077440013276232, 2.0809551104636923, 2.077440013276232, 2.0686522703075743, 2.0721673674950347, 2.0633796245263794, 2.0616220759326493, 2.0528343329639918, 2.0458041385890664, 2.0370163956204115, 2.031743749839216, 2.028228652651754, 2.022956006870561, 2.017683361089369, 2.0088956181207114, 2.0053805209332487, 2.0018654237457887, 2.0001078751520565, 2.0018654237457887, 1.9965927779645936, 1.987805034995936, 1.977259743433551, 1.975502194839821, 1.970229549058626, 1.9579267089025083, 1.9561691603087759, 1.9473814173401207, 1.9403512229651956, 1.9333210285902707, 1.9280483828090755, 1.9192606398404206, 1.9087153482780355, 1.8999276053093779, 1.8999276053093779, 1.884109667965795, 1.8682917306222173, 1.8595039876535597, 1.8454435989037095, 1.834898307341322, 1.8225954671852072, 1.8120501756228167, 1.7979897868729666, 1.7944746896855042, 1.7839293981231163, 1.7751416551544614, 1.7663539121858065, 1.7505359748422236, 1.7470208776547638, 1.7312029403111808, 1.722415197342526, 1.7171425515613308, 1.699567065624018, 1.6855066768741707, 1.6732038367180504, 1.666173642343128, 1.6573858993744703, 1.6468406078120825, 1.6362953162496976, 1.62926512187477, 1.6204773789061149, 1.6134471845311897, 1.6116896359374573, 1.6029018929688048, 1.592356601406417, 1.61520473312492, 1.6837491282804407, 1.7013246142177483, 1.6064169901562673, 1.5695084696879091, 1.5536905323443317, 1.5431452407819417, 1.5431452407819417, 1.5273273034383614, 1.5220546576571663, 1.5273273034383614, 1.523812206250899, 1.523812206250899, 1.5273273034383614, 1.5202971090634363, 1.5325999492195568, 1.5273273034383614, 1.5308424006258214, 1.5431452407819417, 1.544902789375674, 1.5484178865631366, 1.5589631781255242, 1.5695084696879091, 1.5835688584377594, 1.5905990528126872, 1.5976292471876095, 1.6046594415625373, 1.6222349274998475, 1.62926512187477, 1.63981041343716, 1.6591434479682001, 1.6714462881243206, 1.6837491282804407, 1.7030821628114805, 1.7136274543738683, 1.729445391717451, 1.7505359748422236, 1.7663539121858065, 1.7892020439043117, 1.8085350784353542, 1.831383210153857, 1.8524737932786348, 1.8788370221846022, 1.9052002510905728, 1.9315634799965378, 1.961441806089971, 1.987805034995936, 2.026471104058024, 2.0581069787451844, 2.0915004020260795, 2.1284089224944376, 2.1618023457753304, 2.198710866243686, 2.233861838118314, 2.2830731987427813, 2.3270119135860616, 2.379738371398, 2.418404440460088, 2.4711308982720213, 2.532645099052614, 2.5888866540520126, 2.650400854832605, 2.725975444363046, 2.7646415134251336, 2.8243981656119947, 2.9210633382672135, 3.0124558651412365, 3.084515357484215, 3.1706352385770455, 3.262027765451069, 3.3569353895125524, 3.4606307565426935, 3.566083672166567, 3.6662639420092455, 3.7699593090393866, 3.8806848704444525, 3.993167980443254, 4.10213599325459, 4.2111040060659235, 4.3323748590333775, 4.4448579690321735, 4.562613724812167, 4.683884577779619, 4.812185625122, 4.944001769651841, 5.086363205744065, 5.235754836211222, 5.386904015272106, 5.52926545136433, 5.687444824800141, 5.8368364552672976, 5.9967733772968375, 6.30610192979353, 6.478341691979186, 6.643551259789921, 6.808760827600658, 6.965182652442734, 7.137422414628394, 7.29032914228301, 7.492447230562097, 7.636566215248059, 7.747291776653125, 7.900198504307739, 8.067165620712203, 8.197224216648312, 8.429220631020835, 8.585642455862914, 8.749094475079918, 8.949455014765274, 9.075998513513923, 9.239450532730922, 9.40817519772912, 9.559324376790004, 9.675322583976262, 9.866895380692966, 9.9758633935043, 10.13580031553384, 10.293979688969653, 10.429310930686956, 10.59276294990396, 10.649004504903356, 10.823001815682744, 10.90209150240065, 11.049725584274075, 11.228995540834658, 11.366084331145693, 11.508445767237916, 11.642019460361494, 11.768562959110136, 11.905651749421176, 12.065588671450715, 12.241343530823832, 12.371402126759948, 12.585823055195151, 12.606913638319927, 12.867030830192144, 13.185147125657501, 13.396052956905242, 13.603443690965518, 13.83192500815058, 14.789788991734092, 17.011330414210352, 16.030618298908333, 15.981406938283856, 16.07455701375161, 15.802136981723274, 15.800379433129542, 16.00425507000236, 16.248554324531, 16.299523233749206, 16.77757645124409, 17.11151068405303, 16.812727423118723, 17.187085273583474, 16.94630111624229, 17.89713490545088, 18.072889764823994, 17.842650899045214, 17.6563507481097, 17.695016817171783, 17.872529225138642, 17.911195294200724, 17.890104711075956, 18.043011438730566, 17.958649106231476, 18.048284084511764, 18.072889764823994, 18.004345369668485, 18.148464354354438, 18.1801002290416, 18.17131248607295, 18.25040217279085, 18.257432367165777, 18.31367392216517, 18.35058244263353, 18.403308900445467, 18.41561174060159, 18.392763608883076, 18.459550455444862, 18.4841561357571, 18.507004267475608, 18.51930710763173, 18.57203356544366, 18.58960905138097, 18.619487377474403, 18.642335509192907, 18.64936570356783, 18.60718453731829, 18.605426988724552, 18.59839679434963, 18.57730621122485, 18.59488169716217, 18.56500337106873, 18.55797317669381, 18.57027601684993, 18.56676091966247, 18.531609947787846, 18.538640142162766, 18.528094850600382, 18.521064656225455, 18.52985239919411, 18.5122769132568, 18.482398587163367, 18.605426988724552, 18.614214731693213, 18.56148827388127, 18.56500337106873, 18.57203356544366, 18.549185433725157, 18.540397690756503, 18.52985239919411, 18.52985239919411, 18.5122769132568, 18.51403446185053, 18.515792010444265, 18.482398587163367, 18.494701427319487, 18.475368392788447, 18.464823101226052, 18.443732518101285, 18.459550455444862, 18.44900516388247, 18.427914580757704, 
